vi "GetControlName.vi"(6 "error in":errorcluster, 9 "Control in":refnum<class "Control.lvclass">) -> (0 "error out":errorcluster, 3 "Control out":refnum<class "Control.lvclass">, 4 "name":string)   [LabVIEW 2014, in "Raspberry Pi Compatible Compiler for LabVIEW.lvlib" / "PythonConverter_GUI.lvclass"]
uses:
  PythonConverter_GUI.lvclass
  VI Interpreter/Classes/Control/Control.lvclass
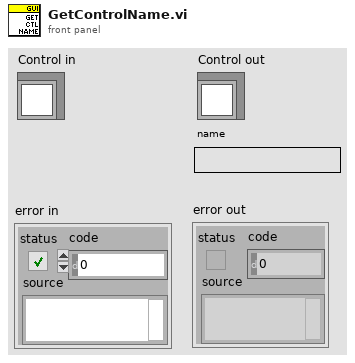
[diagram p1: front panel]
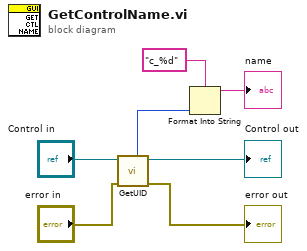
[diagram p0: block diagram]
diagram:
  n1 = call-dynamic "GetUID.vi"("error in"="error in", "GObject in"="Control in") -> ("error out"=→"error out":errorcluster, "GObject out"=→"Control out":refnum<class "Control.lvclass">, "UID"=w2:i32)  [unwired: 5 in]
  n2 = Format Into String(format string="c_%d", w2) -> (resulting string=→"name":string)  [unwired: 2 in, 1 out]
